vi "Get Default VI Resources.vi"(7 "Force reload? (F)":bool, 8 "Error in":errorcluster caption="Error in (no error)") -> (0 "Error out":errorcluster, 3 "Resources":T1)   [LabVIEW 2018, in "Resource Manipulation.lvlib"]
uses:
  Resource Manipulation.lvlib
  Resource Array.ctl
  Resource.ctl
  Blank VI.vi
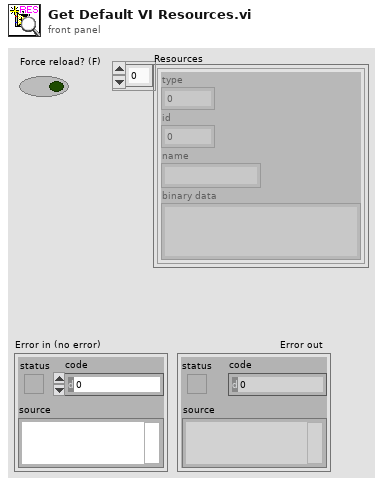
[diagram p1: front panel]
types:
  T1 = typedef "Resource Manipulation.lvlib/Resource Array.ctl" = T2[]
  T2 = typedef "Resource Manipulation.lvlib/Resource.ctl" = cluster{"type":u32, "id":i32, "name":string, "binary data":string}
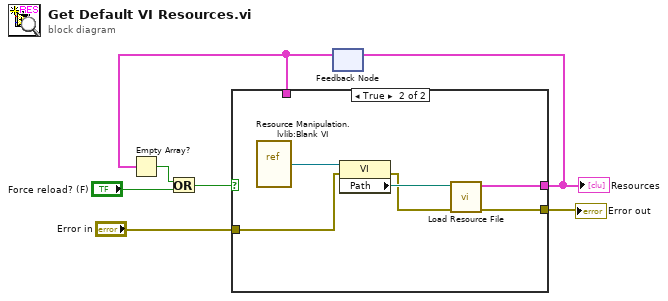
[diagram p0: block diagram]
diagram:
  n1 = feedback #1() -> (w1:T1)  [unwired: 1 in]
  n2 = Empty Array?(array=w1) -> (empty?=w5:bool)
  n3 = Or(x=w5, y="Force reload? (F)") -> (x .or. y?=w3:bool)
  n4 = case shown="True" w3 {
    tunnel: [w9 w13] -> w2
    tunnel: "Error in" -> [w8 w11]
    tunnel: [w8 w10] -> w6
    tunnel: w1 -> [w9 _]
    frame False {
    }
    frame True {
      n5 = vi-ref "Resource Manipulation.lvlib:Blank VI.vi"() -> (w15:refnum<vi>)
      n6 = property class="VI"(reference=w15, error in=w11) -> (error out=w12:errorcluster, "Path"=w14:path)  [unwired: 1 out]
      n7 = call "Load Resource File.vi"("error in (no error)"=w12, "Resource file"=w14) -> ("error out"=w10:errorcluster, "Resources"=w13:T1)  [unwired: 7 in, 1 out]
    }
  }
  "Error out" <- w6
  "Resources" <- w2
  n8 = feedback-in #1(w2) -> ()
